vi "Read class.vi"(8 "error in":errorcluster, 11 "Modbus Slave configuration in":refnum<class "Modbus Module configuration.lvclass">) -> (0 "error out":errorcluster, 2 "class":T1, 3 "Modbus Slave configuration out":refnum<class "Modbus Module configuration.lvclass">)   [LabVIEW 2015, in "Modbus Module configuration.lvclass"]
uses:
  Modbus Module configuration.lvclass
  modbus class.ctl
  Modbus Module configuration.lvclass/Modbus Module configuration.ctl
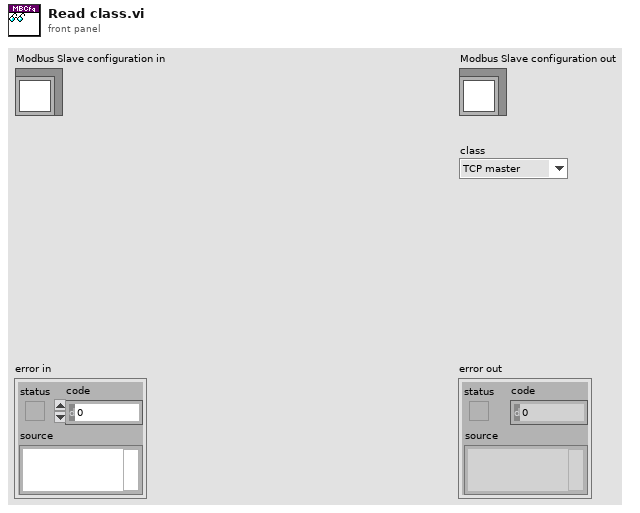
[diagram p1: front panel]
types:
  T1 = typedef "Modbus Module configuration.lvclass/modbus class.ctl" = enum16{"TCP master", "TCP slave", "serial master", "serial slave"}
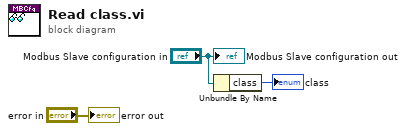
[diagram p0: block diagram]
diagram:
  n1 = Unbundle By Name("Modbus Slave configuration in") -> ("class"=→"class":T1)
  "error out" <- "error in"
  "Modbus Slave configuration out" <- "Modbus Slave configuration in"
